vi "Intersperse Data with Invalid Data 2parallel samples (single channel).vi"(1 "Intersperse Ratio":dbl=0.1, 5 "Channel0 Input":dbl[](array[numeric]) format="%.16g") -> (6 "Channel0 Output":dbl[](array[numeric]), 10 "Data Valid":bool[](array[boolean]))   [LabVIEW 2011]
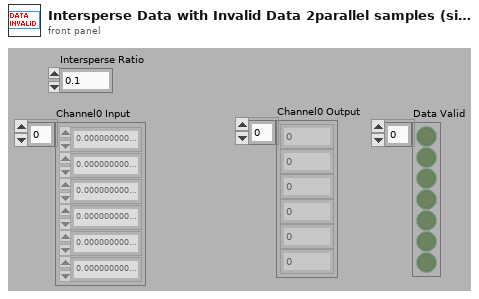
[diagram p1: front panel]
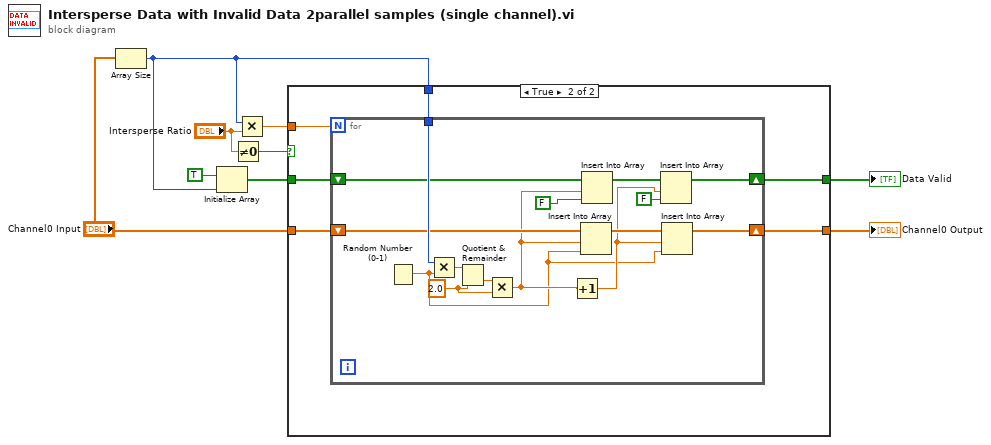
[diagram p0: block diagram]
diagram:
  n1 = Array Size(array="Channel0 Input") -> (size(s)=w8:i32)
  n2 = Initialize Array(TRUE, w8) -> (w6:bool[])
  n3 = Not Equal To 0?(x="Intersperse Ratio") -> (x != 0?=w1:bool)
  n4 = Multiply(x=w8, y="Intersperse Ratio") -> (x*y=w3:dbl)
  n5 = case shown="True" w1 {
    tunnel: "Channel0 Input" -> [w11 w17]
    tunnel: w8 -> [_ w16]
    tunnel: w6 -> [w10 w15]
    tunnel: [w10 w14] -> w5
    tunnel: [w11 w13] -> w4
    tunnel: w3 -> [_ w12]
    frame False {
    }
    frame True {
      n6 = for {
        N: w12 -> [_]
        tunnel: w16 -> [w32]
        shift-right: [w22] -> w13
        shift-left: w17 -> [w31]
        shift-right: [w24] -> w14
        shift-left: w15 -> [w30]
        w26 = 2.0 ("y")
        n7 = Random Number (0-1)() -> (number: 0 to 1=w18:dbl)
        n8 = Multiply(x=w32, y=w18) -> (x*y=w28:dbl)
        n9 = Quotient & Remainder(x=w28, y=w26) -> (floor(x/y)=w27:dbl)  [unwired: 1 out]
        n10 = Multiply(x=w27, y=w26) -> (x*y=w21:dbl)
        n11 = Increment(x=w21) -> (x+1=w20:dbl)
        n12 = Insert Into Array(array=w31, index=w21, new element=w18) -> (w23:dbl[])
        n13 = Insert Into Array(array=w30, index=w21, new element=FALSE) -> (w25:bool[])
        n14 = Insert Into Array(array=w25, index=w20, new element=FALSE ("new element/subarray")) -> (w24:bool[])
        n15 = Insert Into Array(array=w23, index=w20, new element=w18) -> (w22:dbl[])
      }
    }
  }
  "Data Valid" <- w5
  "Channel0 Output" <- w4
